vi "same.vi"(8 "error in (no error)":errorcluster, 10 "Name":string, 11 "Category in":refnum<class "Category.lvclass">) -> (0 "error out":errorcluster, 2 "Equals?":bool, 3 "Category out":refnum<class "Category.lvclass">)   [LabVIEW 2020, in "Category.lvclass"]
uses:
  Category.lvclass
  Category.lvclass/Category.ctl
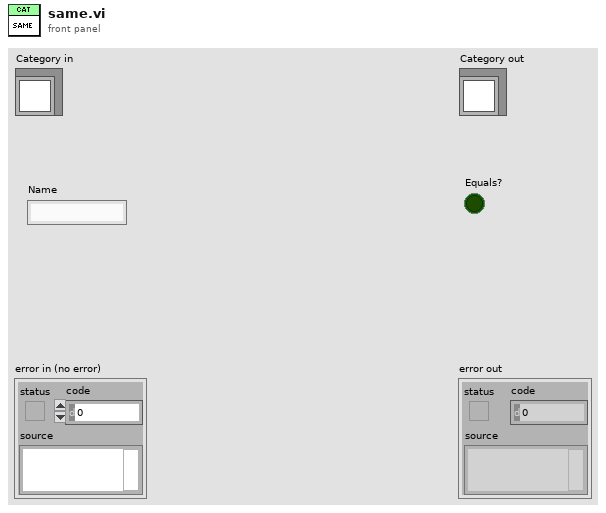
[diagram p1: front panel]
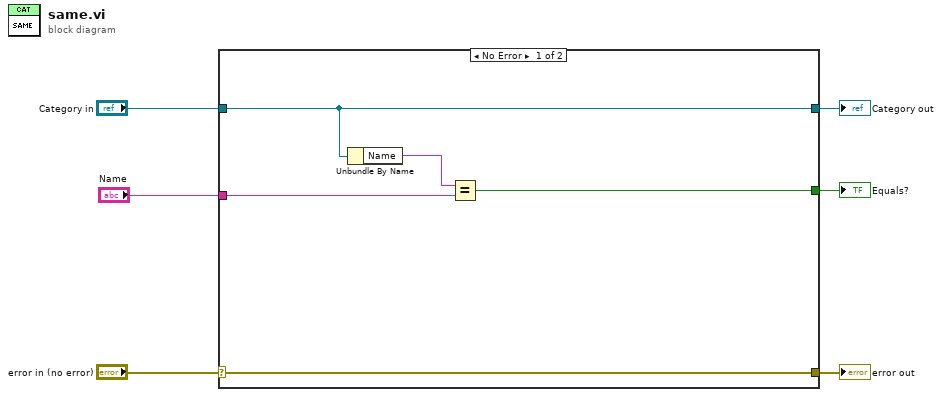
[diagram p0: block diagram]
diagram:
  n1 = case shown="No Error" "error in (no error)" {
    selector: "error in (no error)" -> [w11 w13]
    tunnel: [w11 w13] -> w5
    tunnel: [w10 w12] -> w3
    tunnel: "Category in" -> [w10 w12]
    tunnel: [w8 _] -> w2
    tunnel: "Name" -> [w7 _]
    frame No Error {
      n2 = Unbundle By Name(w10) -> ("Name"=w9:string)
      n3 = Equal?(x=w9, y=w7) -> (x = y?=w8:bool)
    }
    frame Error {
    }
  }
  "error out" <- w5
  "Category out" <- w3
  "Equals?" <- w2
